vi "SaveSetup.vi"(0 "Pegs":refnum<vi>, 1 "Rings Rej":refnum<vi>, 2 "Pegs Left":refnum<vi>, 5 "Rings":refnum<vi>, 7 "RingQ":refnum<vi>, 9 "No Assem":refnum<vi>, 11 "Pegs Rej":refnum<vi>, 12 "Total Rej":refnum<vi>, 13 "Rings Left":refnum<vi>) -> (4 "Path":path)   [LabVIEW 2016]
uses:
  <vilib>/Utility/sysdir.llb/System Directory Type.ctl
  <vilib>/Utility/file.llb/Read Delimited Spreadsheet (string).vi
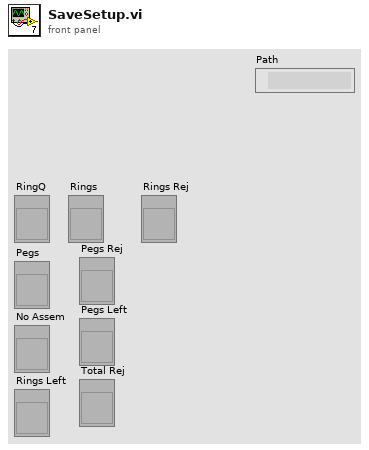
[diagram p1: front panel]
types:
  T1 = enum16{"open", "replace", "create", "open or create", "replace or create", "replace or create with confirmation"}
  T2 = typedef "System Directory Type.ctl" = i32
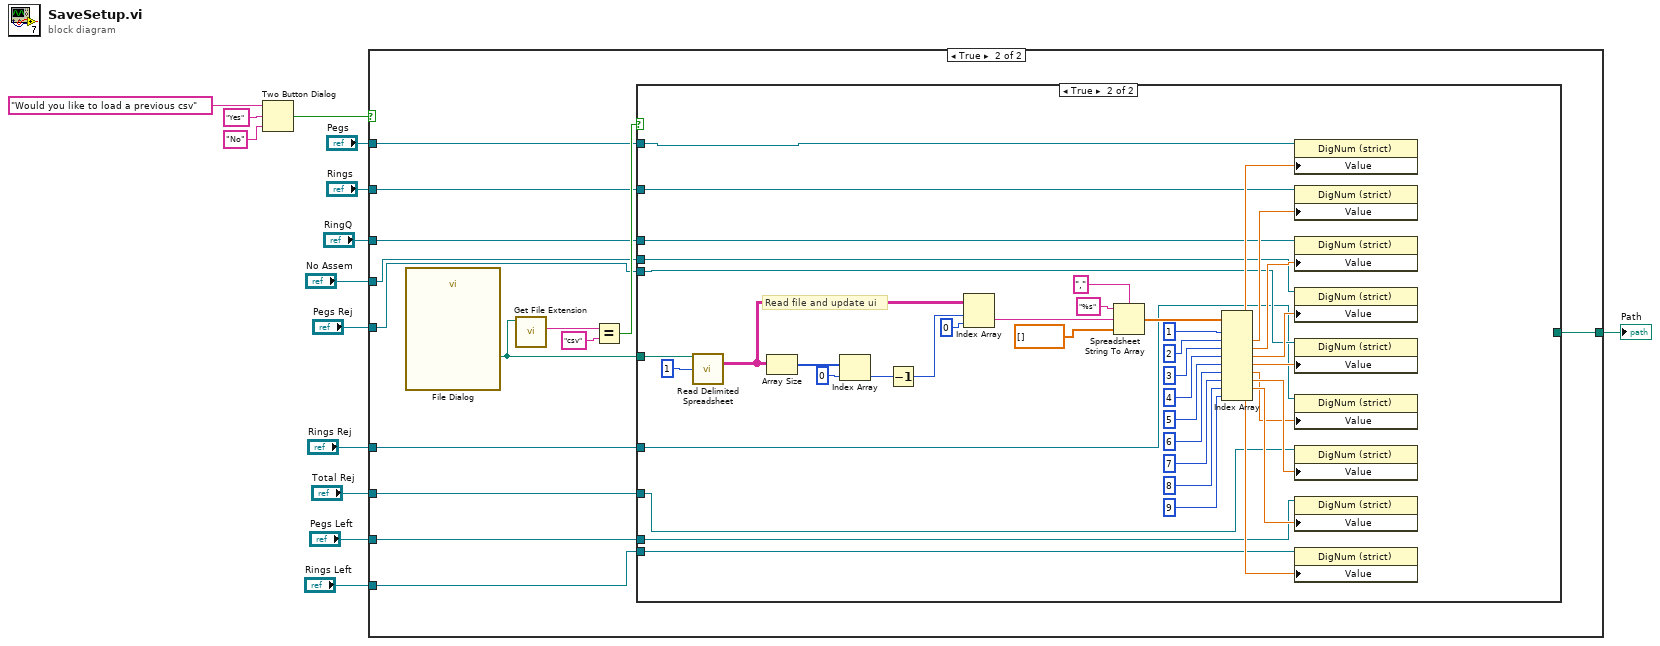
[diagram p0: block diagram]
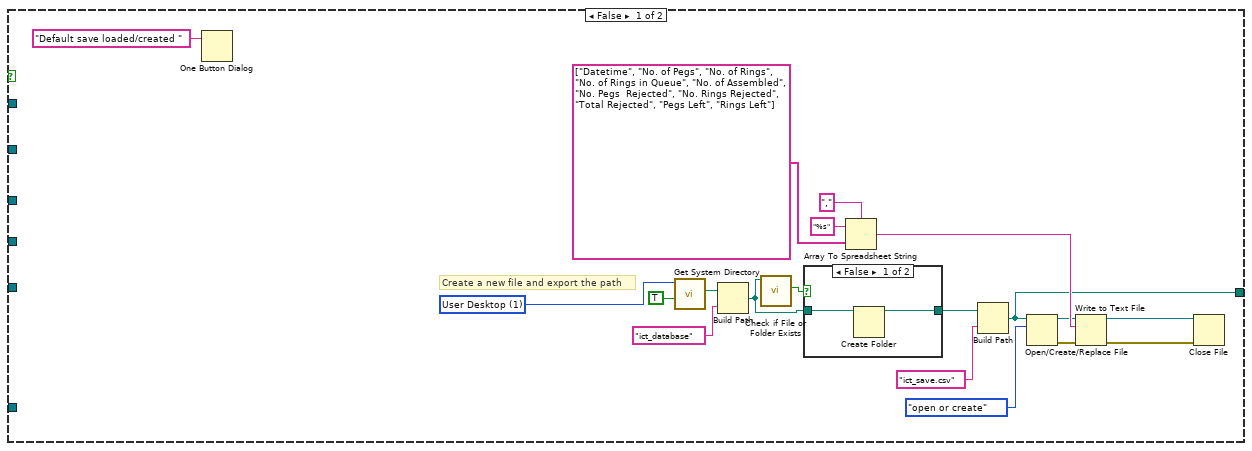
[diagram p2: hidden frame]
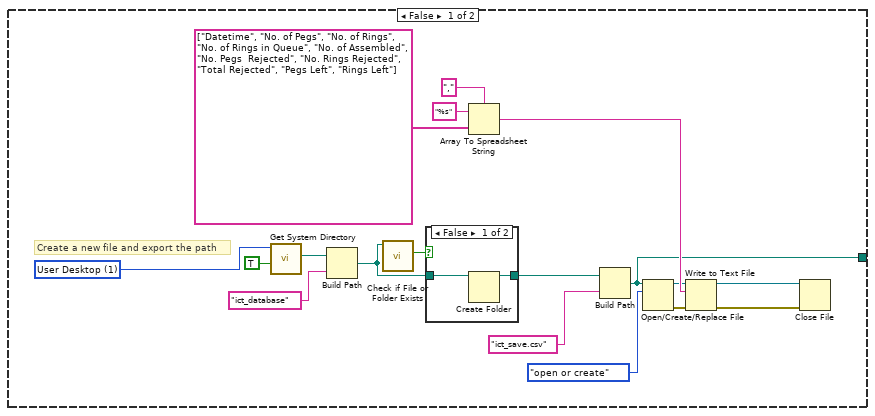
[diagram p4: hidden frame]
diagram:
  n1 = Two Button Dialog(message="Would you like to load a previous csv", 1:"No" ("F button name (\"Cancel\")"), 2:"Yes" ("T button name (\"OK\")")) -> (T button?=w13:bool)
  n2 = case shown="True" w13 {
    tunnel: [w17 w46] -> w14
    tunnel: "Pegs" -> [_ w45]
    tunnel: "Rings" -> [_ w44]
    tunnel: "RingQ" -> [_ w43]
    tunnel: "No Assem" -> [_ w42]
    tunnel: "Pegs Rej" -> [_ w41]
    tunnel: "Rings Rej" -> [_ w40]
    tunnel: "Total Rej" -> [_ w39]
    tunnel: "Pegs Left" -> [_ w38]
    tunnel: "Rings Left" -> [_ w37]
    frame False {
      w27 = T2 1 items=["User Home"=0, "User Desktop"=1, "User Documents"=2, "User Application Data"=3, "User Preferences"=4, "User Temporary"=5, "Public Documents"=6, "Public Application Data"=7, "Public Preferences"=8, "Public Cache"=13, "System Core Libraries"=9, "System Installed Libraries"=10, "Application Files"=11, "Boot Volume Root"=12] ("system directory type")
      # "Create a new file and export the path"
      n3 = One Button Dialog(message="Default save loaded/created ") -> ()  [unwired: 1 in, 1 out]
      n4 = call <vilib>:"Get System Directory.vi"("create directory if not found? (F)"=TRUE, "system directory type"=w27) -> ("system directory"=w28:path)  [unwired: 9 in]
      n5 = Build Path(base path=w28, name or relative path="ict_database") -> (appended path=w31:path)
      n6 = call <vilib>:"Check if File or Folder Exists.vi"("path"=w31) -> ("file or folder exists?"=w30:bool)  [unwired: 8 in, 2 out]
      n7 = case shown="False" w30 {
        tunnel: w31 -> [w35 w36]
        tunnel: [w34 w36] -> w32
        frame False {
          n8 = Create Folder(path (use dialog)=w35) -> (created path=w34:path)  [unwired: 2 in, 2 out]
        }
        frame True {
        }
      }
      n9 = Array To Spreadsheet String(delimiter (Tab)=",", array=string[] ["Datetime", "No. of Pegs", "No. of Rings", "No. of Rings in Queue", "No. of Assembled", "No. Pegs  Rejected", "No. Rings Rejected", "Total Rejected", "Pegs Left", "Rings Left"], 3:"%s" ("format string")) -> (spreadsheet string=w22:string)
      n10 = Build Path(base path=w32, name or relative path="ict_save.csv") -> (appended path=w17:path)
      n11 = Open/Create/Replace File(file path (use dialog)=w17, operation (0:open)=T1."open or create") -> (refnum out=w20:refnum<file>, error out=w21:errorcluster)  [unwired: 4 in, 1 out]
      n12 = Write to Text File(file (use dialog)=w20, text=w22, error in=w21) -> (refnum out=w19:refnum<file>, error out=w18:errorcluster)  [unwired: 1 in, 1 out]
      n13 = Close File(refnum=w19, error in=w18) -> ()  [unwired: 2 out]
    }
    frame True {
      n14 = call "File Dialog"() -> ("selected path"=w47:path)  [unwired: 12 in, 3 out]
      n15 = call <vilib>:"Get File Extension.vi"("file"=w47) -> ("lowercase file extension"=w50:string)  [unwired: 6 in, 4 out]
      n16 = Equal?(x=w50, y="csv") -> (x = y?=w48:bool)
      n17 = case shown="True" w48 {
        tunnel: w47 -> [_ w107]
        tunnel: [w52 _] -> w46
        tunnel: w45 -> [_ w80]
        tunnel: w44 -> [_ w79]
        tunnel: w43 -> [_ w78]
        tunnel: w42 -> [_ w77]
        tunnel: w41 -> [_ w76]
        tunnel: w40 -> [_ w75]
        tunnel: w39 -> [_ w74]
        tunnel: w38 -> [_ w73]
        tunnel: w37 -> [_ w72]
        frame False {
          w62 = T2 1 items=["User Home"=0, "User Desktop"=1, "User Documents"=2, "User Application Data"=3, "User Preferences"=4, "User Temporary"=5, "Public Documents"=6, "Public Application Data"=7, "Public Preferences"=8, "Public Cache"=13, "System Core Libraries"=9, "System Installed Libraries"=10, "Application Files"=11, "Boot Volume Root"=12] ("system directory type")
          # "Create a new file and export the path"
          n18 = call <vilib>:"Get System Directory.vi"("create directory if not found? (F)"=TRUE, "system directory type"=w62) -> ("system directory"=w63:path)  [unwired: 9 in]
          n19 = Build Path(base path=w63, name or relative path="ict_database") -> (appended path=w66:path)
          n20 = call <vilib>:"Check if File or Folder Exists.vi"("path"=w66) -> ("file or folder exists?"=w65:bool)  [unwired: 8 in, 2 out]
          n21 = case shown="False" w65 {
            tunnel: w66 -> [w70 w71]
            tunnel: [w69 w71] -> w67
            frame False {
              n22 = Create Folder(path (use dialog)=w70) -> (created path=w69:path)  [unwired: 2 in, 2 out]
            }
            frame True {
            }
          }
          n23 = Array To Spreadsheet String(delimiter (Tab)=",", array=string[] ["Datetime", "No. of Pegs", "No. of Rings", "No. of Rings in Queue", "No. of Assembled", "No. Pegs  Rejected", "No. Rings Rejected", "Total Rejected", "Pegs Left", "Rings Left"], 3:"%s" ("format string")) -> (spreadsheet string=w57:string)
          n24 = Build Path(base path=w67, name or relative path="ict_save.csv") -> (appended path=w52:path)
          n25 = Open/Create/Replace File(file path (use dialog)=w52, operation (0:open)=T1."open or create") -> (refnum out=w55:refnum<file>, error out=w56:errorcluster)  [unwired: 4 in, 1 out]
          n26 = Write to Text File(file (use dialog)=w55, text=w57, error in=w56) -> (refnum out=w53:refnum<file>, error out=w54:errorcluster)  [unwired: 1 in, 1 out]
          n27 = Close File(refnum=w53, error in=w54) -> ()  [unwired: 2 out]
        }
        frame True {
          # "Read file and update ui"
          n28 = call-poly <vilib>:"Read Delimited Spreadsheet.vi"("file path (dialog if empty)"=w107, "start of read offset (chars.:0)"=1) -> ("all rows"=w106:string[][])  [unwired: 8 in, 5 out]
          n29 = Array Size(array=w106) -> (size(s)=w109:i32[])
          n30 = Index Array(array=w109, index=0) -> (element=w111:i32)
          n31 = Decrement(x=w111) -> (x-1=w105:i32)
          n32 = Index Array(array=w106, index (row)=w105, index (col)=0 ("disabled index (col)")) -> (element=w103:string)
          n33 = Spreadsheet String To Array(delimiter (Tab)=",", format string="%s", spreadsheet string=w103, array type (2D Dbl)=dbl[] []) -> (array=w100:dbl[])
          n34 = Index Array(array=w100, index #1=1 ("index"), index #2=2 ("index"), index #3=3 ("index"), index #4=4 ("index"), index #5=5 ("index"), index #6=6 ("index"), index #7=7 ("index"), index #8=8 ("index"), index #9=9 ("index")) -> (element #1=w89:dbl, element #2=w81:dbl, element #3=w82:dbl, element #4=w83:dbl, element #5=w84:dbl, element #6=w85:dbl, element #7=w87:dbl, element #8=w86:dbl, element #9=w88:dbl)
          n35 = property class="DigNum (strict)"(reference=w80, "Value"=w89) -> ()  [unwired: 1 in, 2 out]
          n36 = property class="DigNum (strict)"(reference=w79, "Value"=w81) -> ()  [unwired: 1 in, 2 out]
          n37 = property class="DigNum (strict)"(reference=w78, "Value"=w82) -> ()  [unwired: 1 in, 2 out]
          n38 = property class="DigNum (strict)"(reference=w77, "Value"=w83) -> ()  [unwired: 1 in, 2 out]
          n39 = property class="DigNum (strict)"(reference=w76, "Value"=w84) -> ()  [unwired: 1 in, 2 out]
          n40 = property class="DigNum (strict)"(reference=w75, "Value"=w85) -> ()  [unwired: 1 in, 2 out]
          n41 = property class="DigNum (strict)"(reference=w74, "Value"=w87) -> ()  [unwired: 1 in, 2 out]
          n42 = property class="DigNum (strict)"(reference=w73, "Value"=w86) -> ()  [unwired: 1 in, 2 out]
          n43 = property class="DigNum (strict)"(reference=w72, "Value"=w88) -> ()  [unwired: 1 in, 2 out]
        }
      }
    }
  }
  "Path" <- w14
